vi "ztscopeM Input External.vi"(8 "error in":errorcluster, 9 "Impedance":dbl(ring)=50.0 items=["50 Ohm"=50.0, "1 MOhm"=1000000.0], 10 "Level":dbl, 11 "Instrument Handle In":i32) -> (0 "error out":errorcluster, 3 "Instrument Handle Out":i32)   [LabVIEW 2013]
doc: "Configure the external input settings.."
uses:
  ztscopeM.dll
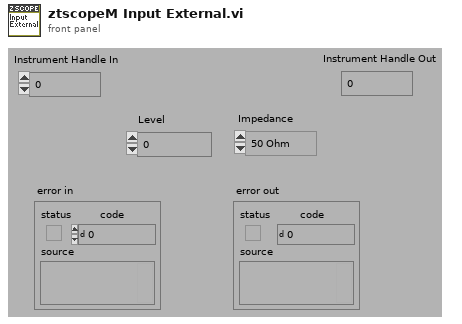
[diagram p1: front panel]
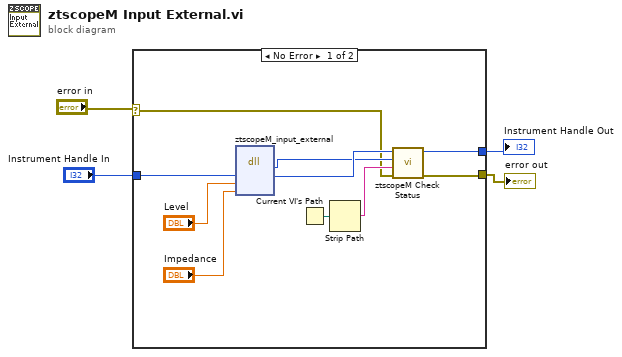
[diagram p0: block diagram]
diagram:
  n1 = case shown="No Error" "error in" {
    selector: "error in" -> [w7 w16]
    tunnel: [w5 w16] -> w1
    tunnel: "Instrument Handle In" -> [w14 w15]
    tunnel: [w6 w15] -> w3
    frame No Error {
      n2 = dll-call lib="C:/Program Files/National Instruments/instr.lib/ztscopem/ztscopeM.dll" fn="ztscopeM_input_external"("instrumentHandle"=w14, "level"="Level", "impedance"="Impedance") -> (w8:i32, "instrumentHandle"=w9:i32)  [unwired: 5 in, 2 out]
      n3 = Current VI's Path() -> (path=w11:path)
      n4 = Strip Path(path=w11) -> (name=w10:string)  [unwired: 1 out]
      n5 = call "ztscopeM Check Status.vi"("error in"=w7, "name of VI"=w10, "status"=w8, "instrument handle in"=w9) -> ("error out"=w5:errorcluster, "instrument handle out"=w6:i32)  [unwired: 2 in]
    }
    frame Error {
    }
  }
  "Instrument Handle Out" <- w3
  "error out" <- w1
